vi "MX 模块测试.vi"() -> ()   [LabVIEW 2012]
uses:
  Component Assemble Input.ctl
  State Assemble.ctl
  Single State.ctl
  Group State.ctl
  MX Operation Options.ctl
  <vilib>/Utility/file.llb/Read From Spreadsheet File (string).vi
panel:
  in  "基路径":path
  in  "选项卡控件":enum32{"选项卡 1", "选项卡 2"}(tab)
  in  "批量执行":bool
  in  "执行":bool
  in  "input/output":bool
  in  "停止按钮":bool
  in  "Component Assemble Input":T1
  out "State Assemble":T2
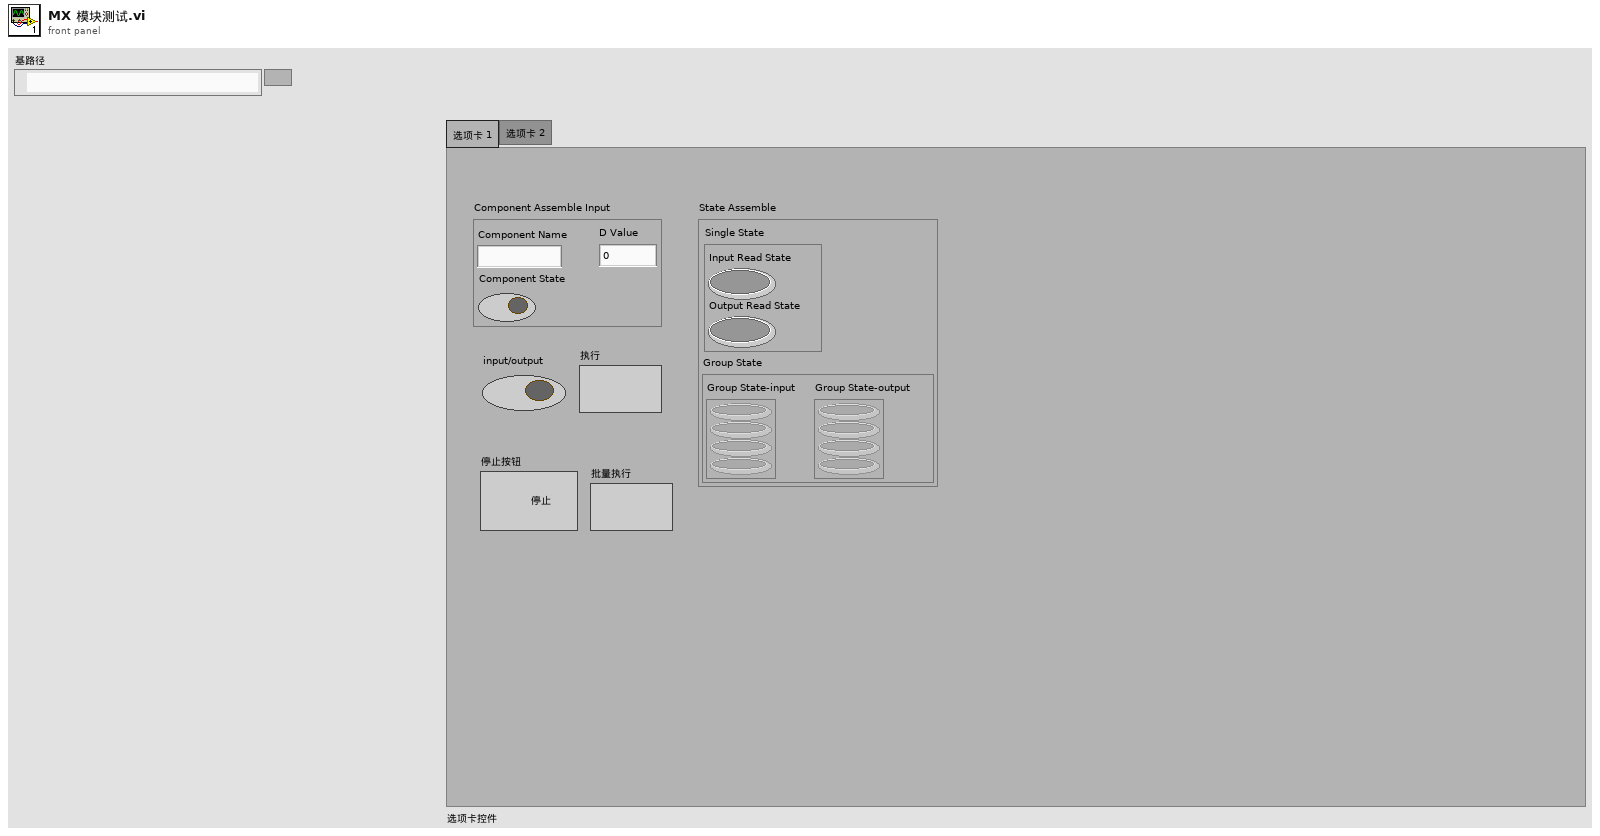
[diagram p1: front panel]
types:
  T1 = typedef "Component Assemble Input.ctl" = cluster{"Component Name":string, "Component State":bool, "D Value":dbl}
  T2 = typedef "State Assemble.ctl" = cluster{"Single State":T3, "Group State":T4}
  T3 = typedef "Single State.ctl" = cluster{"Input Read State":bool, "Output Read State":bool}
  T4 = typedef "Group State.ctl" = cluster{"Group State-input":bool[], "Group State-output":bool[]}
  T5 = typedef "MX Operation Options.ctl" = enum16{"MX Initial ", "MX Close", "Single component Read", "Single component Write", "Many component Read", "Many component Write", "Load Function Global"}
  T6 = cluster{"String":string, "Component State":bool, "D Value":dbl}
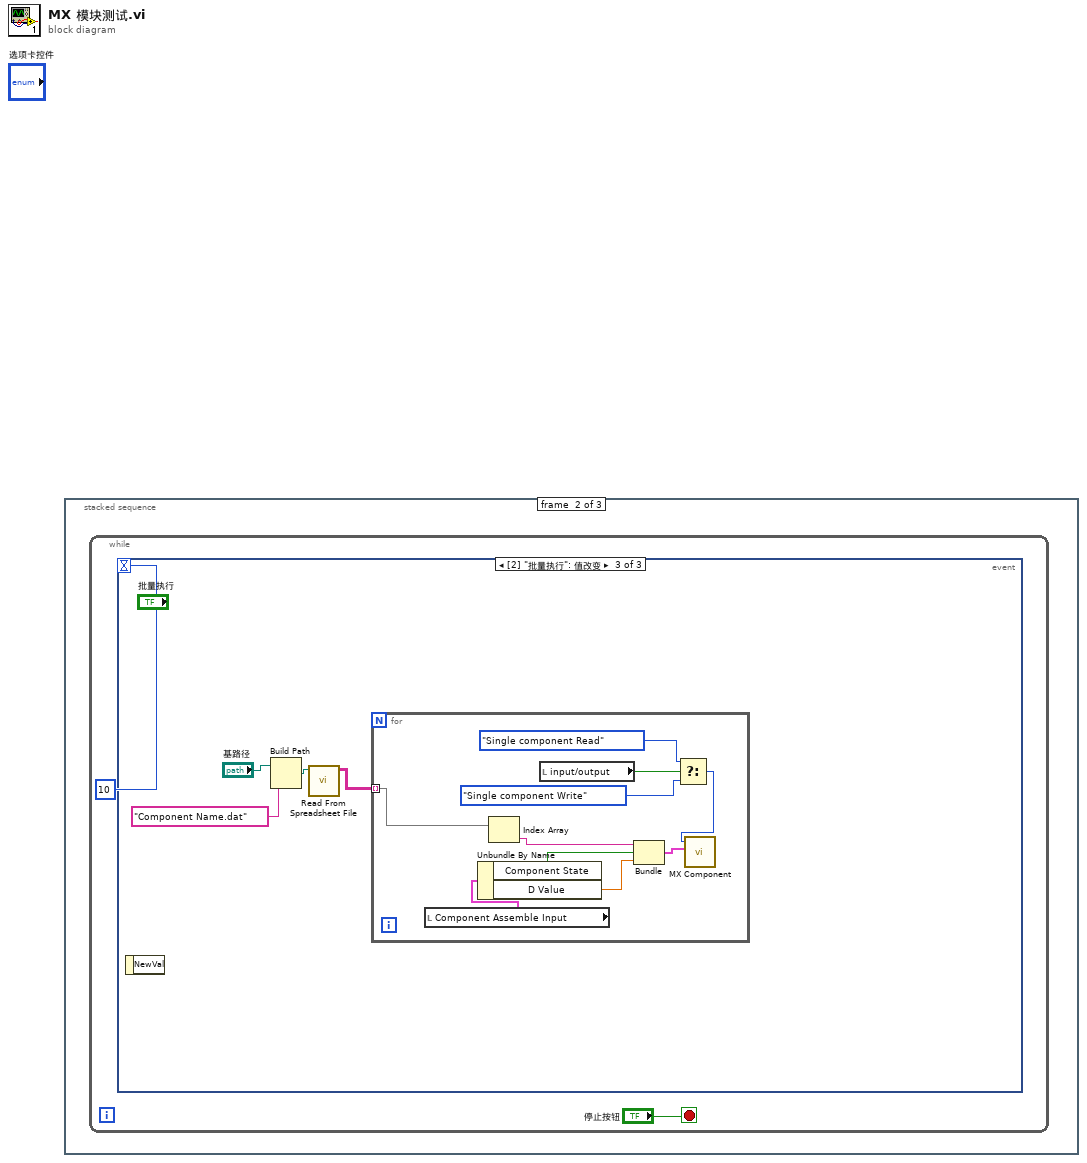
[diagram p0: block diagram]
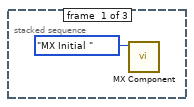
[diagram p2: hidden frame]
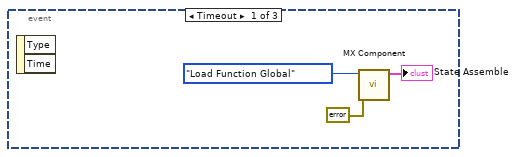
[diagram p3: hidden frame]
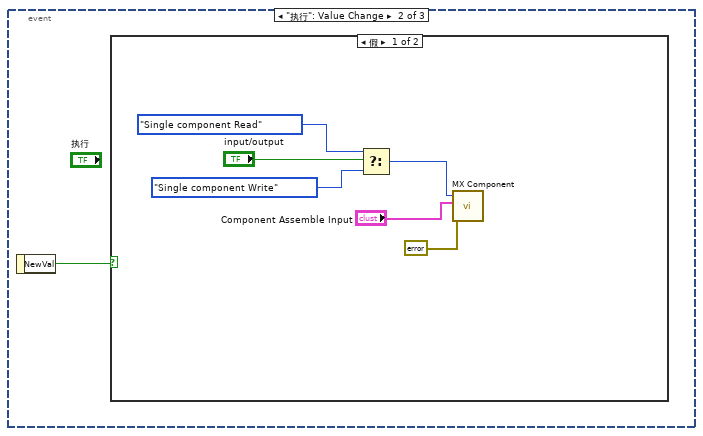
[diagram p4: hidden frame]
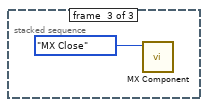
[diagram p6: hidden frame]
diagram:
  n1 = stacked-sequence {
    frame #0 {
      n2 = call "MX Component.vi"("MX Operation Options"=MX_Operation_Options."MX Initial ") -> ()  [unwired: 9 in, 2 out]
    }
    frame #1 {
      n3 = while {
        stop <- "停止按钮" stop-if-true
        n4 = event shown="[2] \"批量执行\": 值改变" {
          selector: _ -> [_ _ _]
          dyn-events: _ -> [_ _ _]
          timeout: 10 -> [_ _ _]
          event Timeout {
            n5 = event-data() -> ()  [unwired: 1 in, 2 out]
            n6 = call "MX Component.vi"("错误输入"=errorcluster {"status"=FALSE, "code"=0, "source"=""}, "MX Operation Options"=MX_Operation_Options."Load Function Global") -> ("State Assemble"=→"State Assemble":T2)  [unwired: 8 in, 1 out]
          }
          event "执行": Value Change {
            n7 = event-data() -> ("NewVal"=w7:bool)  [unwired: 1 in]
            n8 = case shown="假" w7 {
              frame False {
                n9 = Select(t=MX_Operation_Options."Single component Read" ("MX Operation Options"), s="input/output", f=MX_Operation_Options."Single component Write" ("MX Operation Options")) -> (s? t:f=w8:T5)
                n10 = call "MX Component.vi"("错误输入"=errorcluster {"status"=FALSE, "code"=0, "source"=""}, "Component Assemble Input"="Component Assemble Input", "MX Operation Options"=w8) -> ()  [unwired: 7 in, 2 out]
              }
              frame True {
              }
            }
          }
          event "批量执行": Value Change {
            n11 = event-data() -> ()  [unwired: 1 in, 1 out]
            n12 = Build Path(base path="基路径", name or relative path="Component Name.dat" ("名称或相对路径")) -> (appended path=w15:path)
            n13 = call-poly <vilib>:"Read From Spreadsheet File.vi"("file path (dialog if empty)"=w15) -> ("all rows"=w14:string[][])  [unwired: 6 in, 4 out]
            n14 = for {
              tunnel: w14 -> [w27] mode=indexing
              n15 = local read "Component Assemble Input"() -> (w18:T1)
              n16 = Unbundle By Name(w18) -> ("Component State"=w25:bool, "D Value"=w24:dbl)
              n17 = Index Array(array=w27) -> (element=w26:string)  [unwired: 1 in]
              n18 = local read "input/output"() -> (w22:bool)
              n19 = Bundle("String"=w26, "Component State"=w25, "D Value"=w24) -> (w23:T6)  [unwired: 1 in]
              n20 = Select(t=MX_Operation_Options."Single component Read" ("MX Operation Options"), s=w22, f=MX_Operation_Options."Single component Write" ("MX Operation Options")) -> (s? t:f=w21:T5)
              n21 = call "MX Component.vi"("Component Assemble Input"=w23, "MX Operation Options"=w21) -> ()  [unwired: 8 in, 2 out]
            }
          }
        }
      }
    }
    frame #2 {
      n22 = call "MX Component.vi"("MX Operation Options"=MX_Operation_Options."MX Close") -> ()  [unwired: 9 in, 2 out]
    }
  }
